vi "GA Send Eth To Uart String.vi"(8 "error in (no error)":errorcluster caption="错误输入（无错误）", 9 "nLength":i16, 10 "pSendBuf":string, 11 "nUartNum":i16) -> (0 "error out":errorcluster caption="错误输出", 2 "pSendBuf out":string, 3 "function return":i32)   [LabVIEW 2015, in "GAS.lvlib"]
doc: "extern \"C\" __declspec(dllimport) int GA_SendEthToUartString(short nUartNum,unsigned char*pSendBuf, short nLength);"
uses:
  <userlib>/BP_GAS/GAS.lvlib
  <userlib>/BP_GAS/GAS.dll
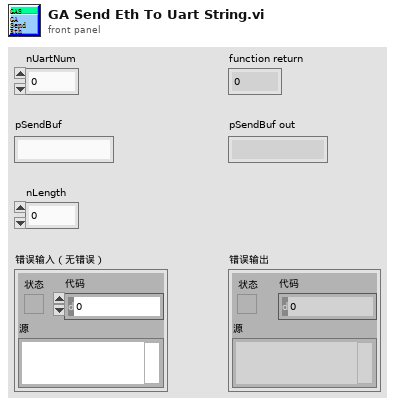
[diagram p1: front panel]
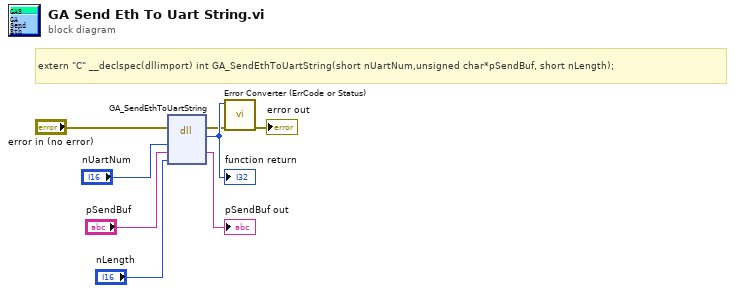
[diagram p0: block diagram]
diagram:
  # "extern \"C\" __declspec(dllimport) int GA_SendEthToUartString(short nUartNum,unsigned char*pSendBuf, short nLength);"
  n1 = dll-call lib="E:/Program Files (x86)/National Instruments/LabVIEW 2015/user.lib/BP_GAS/GAS.*" fn="GA_SendEthToUartString"(error in="error in (no error)", "nUartNum"="nUartNum", "pSendBuf"="pSendBuf", "nLength"="nLength") -> (error out=w2:errorcluster, w8:i32, "pSendBuf"=→"pSendBuf out":string)  [unwired: 4 in, 1 out]
  "function return" <- w8
  n2 = call "Error Converter (ErrCode or Status).vi"("error in (no error)"=w2, "error code"=w8) -> ("error out"=→"error out":errorcluster)  [unwired: 9 in]
